vi "Run.vi"(7 "Team Index":i32, 8 "Column":i32, 9 "Row":i32, 10 "View":i32[](array[numeric]) caption="View (Team Index, -1: empty)", 11 "SquareA In":refnum<class "Ant Mound.lvclass">) -> (0 "Replicated":refnum<class "Square.lvclass">, 1 "Direction":T1, 2 "Action":T2, 3 "Square Out":refnum<class "Square.lvclass">)   [LabVIEW 2017, in "Ant Mound.lvclass"]
uses:
  Ant Mound.lvclass
  C:/GIT/Endigit/SquareBattle/Square/Square.lvclass
  Square/Square.lvclass
  Type Defs/Action Enum.ctl
  Type Defs/Direction Enum.ctl
  Ant Mound.lvclass/Ant Mound.ctl
  DS Square Library/DS Square.lvlib
  Common/Common.lvlib
  Type Defs/SB Type Defs.lvlib
panel:
  # "NW\nN\nNE\nE\nSE\nS\nSW\nW"
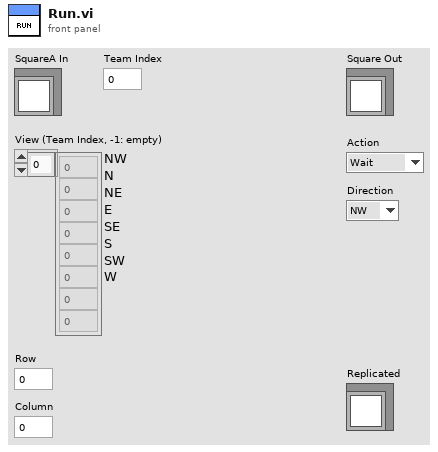
[diagram p1: front panel]
types:
  T1 = typedef "SB Type Defs.lvlib/Direction Enum.ctl" = enum16{"NW", "N", "NE", "E", "SE", "S", "SW", "W"}
  T2 = typedef "SB Type Defs.lvlib/Action Enum.ctl" = enum16{"Wait", "Move", "Attack", "Replicate"}
  T3 = typedef "Common.lvlib/Map DVR.ctl" = refnum<data-value>
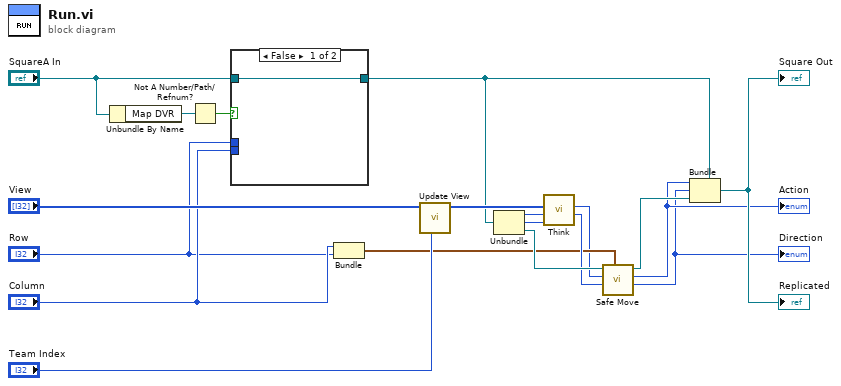
[diagram p0: block diagram]
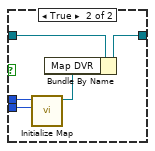
[diagram p2: hidden frame]
diagram:
  n1 = Unbundle By Name("SquareA In") -> ("Map DVR"=w15:T3)
  n2 = Not A Number/Path/Refnum?(number/path/refnum=w15) -> (NaN/Path/Refnum?=w16:bool)
  n3 = case shown="False" w16 {
    tunnel: "Column" -> [_ w25]
    tunnel: "Row" -> [_ w24]
    tunnel: "SquareA In" -> [w20 w23]
    tunnel: [w20 w21] -> w10
    frame False {
    }
    frame True {
      n4 = call "Initialize Map.vi"("Column"=w25, "Row"=w24) -> ("Map DVR"=w22:T3)  [unwired: 9 in]
      n5 = Bundle By Name(cluster=w23, "Map DVR"=w22) -> (w21:refnum<class "Ant Mound.lvclass">)
    }
  }
  n6 = Bundle("Column"="Column", "Row"="Row") -> (w5:cluster{"Column":i32, "Row":i32})  [unwired: 1 in]
  n7 = call "Update View.vi"("Team Index"="Team Index", "View"="View") -> ("View out"=w11:i32[])  [unwired: 9 in]
  n8 = Unbundle(w10) -> (w13:T2, w12:T1, w7:T3)
  n9 = call "Think.vi"("Last Direction"=w12, "Last Action"=w13, "View out"=w11) -> ("Direction"=w6:T1, "Action"=w3:T2)  [unwired: 7 in]
  n10 = call "Safe Move.vi"("Position in"=w5, "Direction in"=w6, "Desired Action"=w3, "Map DVR"=w7) -> ("Direction"=w1:T1, "Action"=w2:T2, "Map DVR out"=w4:T3)  [unwired: 4 in, 1 out]
  "Action" <- w2
  "Direction" <- w1
  n11 = Bundle(cluster=w10, w2, w1, w4) -> (→"Square Out" →"Replicated":refnum<class "Ant Mound.lvclass">)
